vi "Construct Menu Button.vi"(8 "Border Offset":i32=1, 9 "Reset Bool on Value Change?":bool=TRUE, 10 "Nested Item Refs":refnum<vi>[](array[refnum]), 11 "Menu Reference":refnum<vi>) -> (3 "MenuButton out":refnum<class "MenuButton.lvclass">)   [LabVIEW 2017, in "MenuButtons.lvlib" / "MenuButton.lvclass"]
uses:
  MenuButton.lvclass
  MenuButton.lvclass/MenuButton.ctl
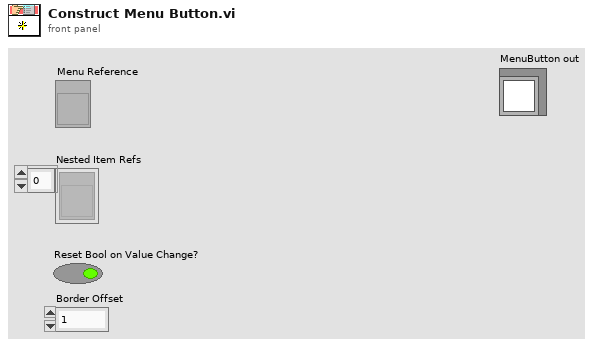
[diagram p1: front panel]
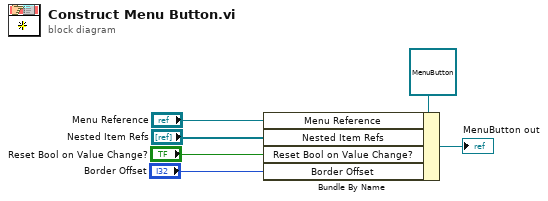
[diagram p0: block diagram]
diagram:
  n1 = Bundle By Name(cluster=refnum<class "MenuButton.lvclass"> refnum ("MenuButton in"), "Menu Reference"="Menu Reference", "Nested Item Refs"="Nested Item Refs", "Reset Bool on Value Change?"="Reset Bool on Value Change?", "Border Offset"="Border Offset") -> (→"MenuButton out":refnum<class "MenuButton.lvclass">)
